vi "WriteErrorFinal1.vi"(8 "error in (no error)":errorcluster, 11 "Error":string) -> (0 "error out":errorcluster)   [LabVIEW 2024]
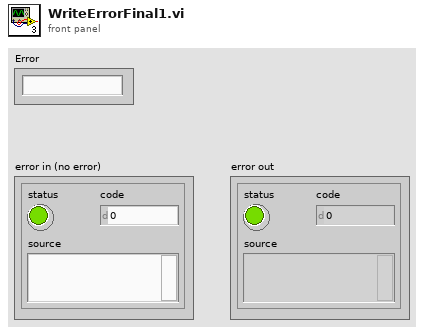
[diagram p1: front panel]
types:
  T1 = enum16{"open", "replace", "create", "open or create", "replace or create", "replace or create with confirmation"}
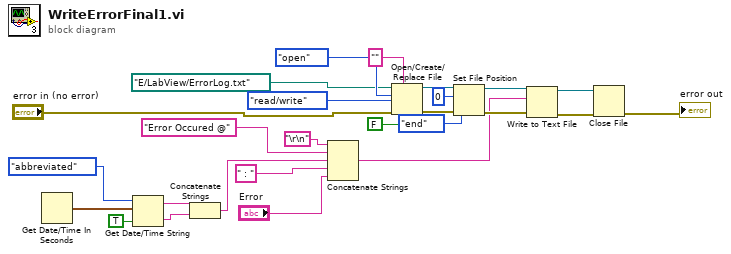
[diagram p0: block diagram]
diagram:
  n1 = Get Date/Time In Seconds() -> (seconds since 1Jan1904=w13:timestamp)
  n2 = Get Date/Time String(date format (0)=enum16{"short", "long", "abbreviated"}."abbreviated", seconds (now)=w13, want seconds? (F)=TRUE) -> (date string=w12:string, time string=w11:string)
  n3 = Concatenate Strings(w12, w11) -> (w10:string)
  n4 = Concatenate Strings("\r\n", "Error Occured @" ("string"), w10, " : " ("string"), "Error") -> (w3:string)
  n5 = Open/Create/Replace File(file path (use dialog)=path "E:/LabView/ErrorLog.txt", error in="error in (no error)", prompt="", operation (0:open)=T1."open", access (0:read/write)=enum16{"read/write", "read-only", "write-only"}."read/write", disable buffering (F)=FALSE) -> (refnum out=w8:refnum<file>, error out=w7:errorcluster)  [unwired: 1 out]
  n6 = Set File Position(offset (in bytes) (0)=i64 0, refnum=w8, from (0:start)=enum16{"start", "end", "current"}."end", error in=w7) -> (refnum out=w5:refnum<file>, error out=w4:errorcluster)
  n7 = Write to Text File(file (use dialog)=w5, text=w3, error in=w4) -> (refnum out=w23:refnum<file>, error out=w24:errorcluster)  [unwired: 1 in, 1 out]
  n8 = Close File(refnum=w23, error in=w24) -> (error out=→"error out":errorcluster)  [unwired: 1 out]
